vi "ConnectDevice.vi"(8 "error in (no error)":errorcluster, 11 "Highland T564 DDG in":refnum<class "Highland T564 DDG.lvclass">) -> (0 "error out":errorcluster, 3 "Highland T564 DDG out":refnum<class "Highland T564 DDG.lvclass">)   [LabVIEW 2020, in "Highland T564 DDG.lvclass"]
doc: "Connect to the phsyical device"
uses:
  Highland T564 DDG.lvclass
  SupportLibraries/DeviceSpecific/HighlandT560Lib/T560SessionClass/T560Session.lvclass
  Highland T564 DDG.lvclass/Highland T564 DDG.ctl
panel:
  out "error out class path":errorcluster
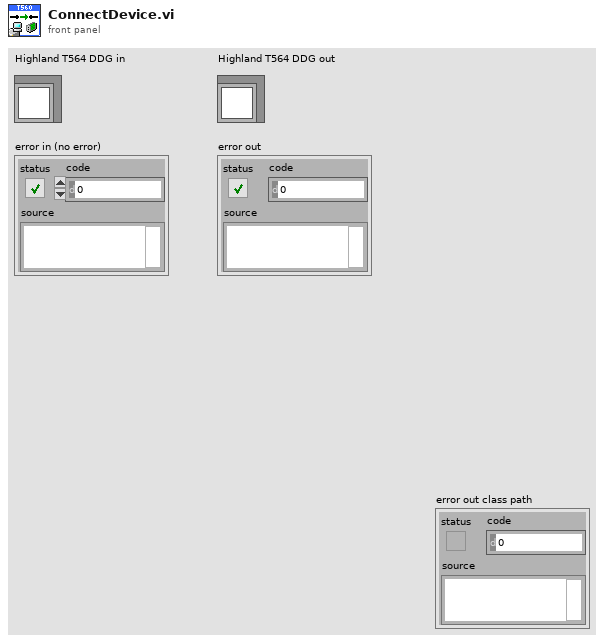
[diagram p1: front panel]
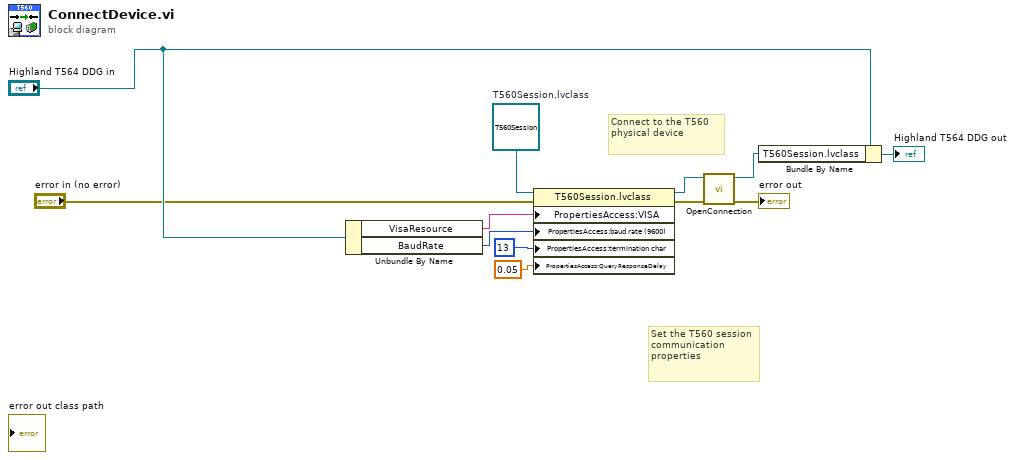
[diagram p0: block diagram]
diagram:
  w1 = refnum<class "T560Session.lvclass"> refnum  # T560Session.lvclass
  # "Connect to the T560 physical device"
  # "Set the T560 session communication properties"
  n1 = Unbundle By Name("Highland T564 DDG in") -> ("VisaResource"=w10:string, "BaudRate"=w11:u32)
  n2 = property class="T560Session.lvclass"(reference=w1, error in="error in (no error)", "PropertiesAccess:VISA"=w10, "PropertiesAccess:baud rate (9600)"=w11, "PropertiesAccess:termination char"=u8 13 ("termination char"), "PropertiesAccess:QueryResponseDelay"=0.05 ("QueryResponseDelay")) -> (reference out=w6:refnum<class "T560Session.lvclass">, error out=w5:errorcluster)
  n3 = call-dynamic "OpenConnection.vi"("error in"=w5, "T560Session in"=w6) -> ("error out"=→"error out":errorcluster, "T560Session out"=w9:refnum<class "T560Session.lvclass">)  [unwired: 8 in]
  n4 = Bundle By Name(cluster="Highland T564 DDG in", "T560Session.lvclass"=w9) -> (→"Highland T564 DDG out":refnum<class "Highland T564 DDG.lvclass">)
